vi "OCV Data to Cluster.vi"(9 "ErrorOutData":T1, 10 "Numeric":i32, 11 "OCVRawData in":T2) -> (3 "OCVRawData out":T2)   [LabVIEW 2019]
uses:
  MeasurementServer_OCVRawData.ctl
  MeasurementServer_ErrorOutData.ctl
  labview-grpc-measurement-server.lvlib
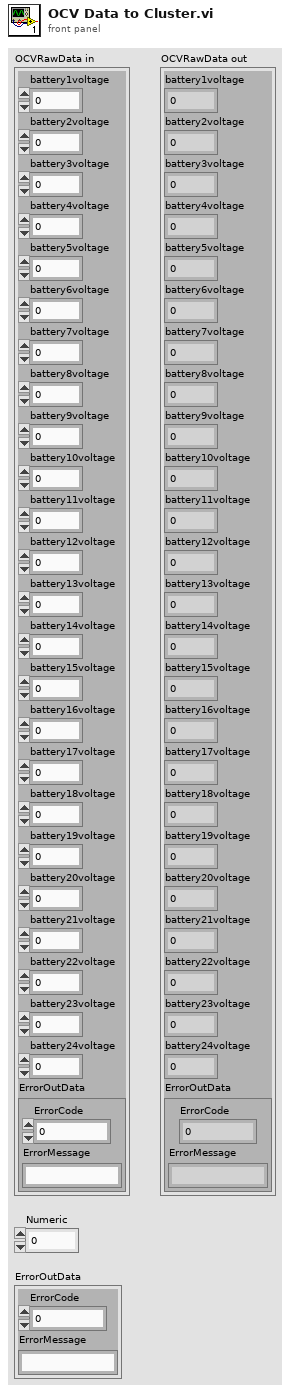
[diagram p1: front panel]
types:
  T1 = typedef "labview-grpc-measurement-server.lvlib/MeasurementServer_ErrorOutData.ctl" = cluster{"ErrorCode":i32, "ErrorMessage":string}
  T2 = typedef "labview-grpc-measurement-server.lvlib/MeasurementServer_OCVRawData.ctl" = cluster{"battery1voltage":dbl, "battery2voltage":dbl, "battery3voltage":dbl, "battery4voltage":dbl, "battery5voltage":dbl, "battery6voltage":dbl, "battery7voltage":dbl, "battery8voltage":dbl, "battery9voltage":dbl, "battery10voltage":dbl, "battery11voltage":dbl, "battery12voltage":dbl, "battery13voltage":dbl, "battery14voltage":dbl, "battery15voltage":dbl, "battery16voltage":dbl, "battery17voltage":dbl, "battery18voltage":dbl, "battery19voltage":dbl, "battery20voltage":dbl, "battery21voltage":dbl, "battery22voltage":dbl, "battery23voltage":dbl, "battery24voltage":dbl, "ErrorOutData":T1}
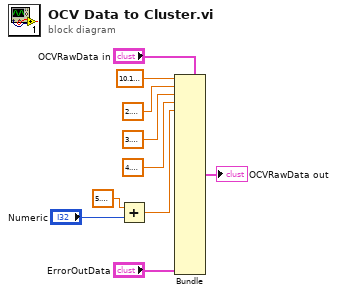
[diagram p0: block diagram]
diagram:
  n1 = Add(x=sgl 5.1 ("Positive Voltage"), y="Numeric") -> (x+y=w8:sgl)
  n2 = Bundle(cluster="OCVRawData in", "battery1voltage"=sgl 10.1 ("Positive Voltage"), "battery2voltage"=sgl 2.1 ("Positive Voltage"), "battery3voltage"=sgl 3.1 ("Positive Voltage"), "battery4voltage"=sgl 4.1 ("Positive Voltage"), "battery5voltage"=w8, "ErrorOutData"="ErrorOutData") -> (→"OCVRawData out":T2)  [unwired: 19 in]
